vi "Vision Research Phantom Series PhCon PhGetExposureRange.vi"(0 "CN in":u32=1, 2 "FrameRate":u32, 5 "Error In (no error)":errorcluster) -> (14 "CN out":u32=1, 16 "pMaxExposure":u32, 17 "pMinExposure":u32, 19 "Error Out":errorcluster)   [LabVIEW 2013, in "VRI.lvlib"]
doc: "PhCon.dll\n\nPhGetExposureRange\nHRESULT PhGetExposureRange(UINT CN, UINT FrameRate, UINT *pMinExposure, UINT *pMaxExposure);\n\nParameters Description\nCN (in) Camera number.\nFrameRate(in) Frame rate.\npMinExposure (out) Pointer to the first result: minimum exposure.\npMaxExposure (out) Pointer to the second result: maximum exposure.\nReturn HRESULT (0=Ok)\nComments Compute the limits of the Exposure parameter for the specified frame rate.\n\nWritten by:\nBLOOMY CONTROLS, INC\nWINDSOR, CT 06095, USA\n860-298-9925\nwww.bloomy.com\nV1.0.0\nMay, 2004"
uses:
  VRI.lvlib
  Phantom DLLs/PhCon.dll
panel:
  # "For instructions on the use of this VI, press Ctrl+H to display the help window and move the mouse over the icon, controls, and indicators"
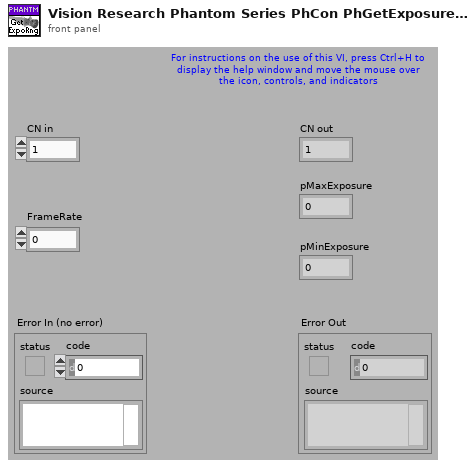
[diagram p1: front panel]
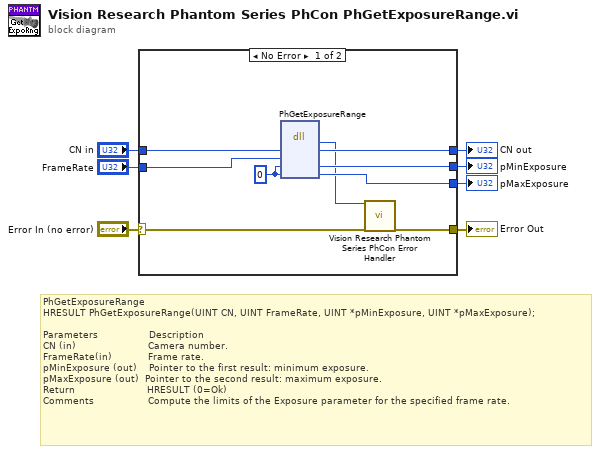
[diagram p0: block diagram]
diagram:
  # "PhGetExposureRange\nHRESULT PhGetExposureRange(UINT CN, UINT FrameRate, UINT *pMinExposure, UINT *pMaxExposure);\n\nParameters                 Description\nCN (in)                        Camera number.\nFrameRate(in)            Frame rate.\npMinExposure (out)    Pointer to the first result: minimum exposure.\npMaxExposure (out)  Pointer to the second result: maximum exposure.\nReturn                        HRESULT (0=Ok)\nComments                  Compute the limits of the Exposure parameter for the specified frame rate."
  n1 = case shown="No Error" "Error In (no error)" {
    selector: "Error In (no error)" -> [w16 w18]
    tunnel: [w15 w18] -> w6
    tunnel: "CN in" -> [w14 w17]
    tunnel: [w13 w17] -> w4
    tunnel: "FrameRate" -> [w12 _]
    tunnel: [w11 _] -> w2
    tunnel: [w10 _] -> w1
    frame No Error {
      w8 = u32 0 ("pMinFrameRate")
      n2 = dll-call lib="C:/Projects/SDK/32-bit/Vision Research Phantom Series Labview Driver/Phantom DLLs/PhCon.dll" fn="PhGetExposureRange"("CN"=w14, "FrameRate"=w12, "pMinExposure"=w8, "pMaxExposure"=w8) -> ("HRESULT"=w9:i32, "CN"=w13:u32, "pMinExposure"=w11:u32, "pMaxExposure"=w10:u32)  [unwired: 4 in, 2 out]
      n3 = call "Vision Research Phantom Series PhCon Error Handler.vi"("ErrNo"=w9, "Error In (no error)"=w16) -> ("Error Out"=w15:errorcluster)  [unwired: 17 out]
    }
    frame Error {
    }
  }
  "Error Out" <- w6
  "CN out" <- w4
  "pMinExposure" <- w2
  "pMaxExposure" <- w1
